vi "TEST ASIC DIGITAL OFFSET GET INIT END.vi"(0 "Min":i32, 1 "Max":i32, 2 "Scaler x":u16[](array[numeric]), 3 "LVDS x":bool[](array[boolean]), 4 "THx":u16[](array[numeric]), 5 "VxLTH":dbl[](array[numeric])) -> (20 "Scaler X min":u16, 21 "Scaler X Max":u16, 22 "LVDS x min":bool, 23 "LVDS X Max":bool, 24 "THX min":u16, 25 "THX Max":u16, 26 "OUT x min":dbl, 27 "OUT x Max":dbl)   [LabVIEW 2019]
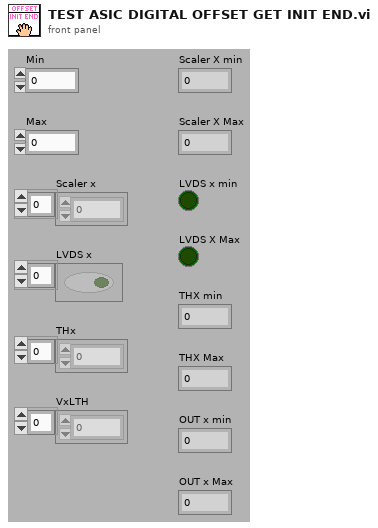
[diagram p1: front panel]
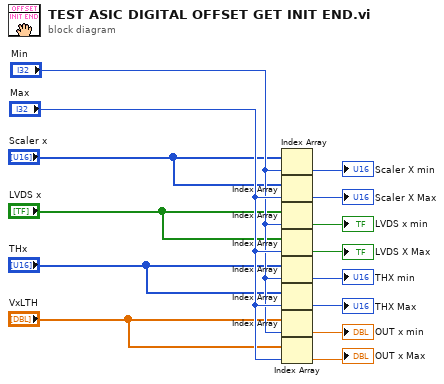
[diagram p0: block diagram]
diagram:
  n1 = Index Array(array="Scaler x", index="Min") -> (element=→"Scaler X min":u16)
  n2 = Index Array(array="Scaler x", index="Max") -> (element=→"Scaler X Max":u16)
  n3 = Index Array(array="LVDS x", index="Min") -> (element=→"LVDS x min":bool)
  n4 = Index Array(array="LVDS x", index="Max") -> (element=→"LVDS X Max":bool)
  n5 = Index Array(array="THx", index="Min") -> (element=→"THX min":u16)
  n6 = Index Array(array="THx", index="Max") -> (element=→"THX Max":u16)
  n7 = Index Array(array="VxLTH", index="Min") -> (element=→"OUT x min":dbl)
  n8 = Index Array(array="VxLTH", index="Max") -> (element=→"OUT x Max":dbl)
